vi "Main.vi"() -> ()   [LabVIEW 2019]
uses:
  <vilib>/addons/Biomedical/Controls/Biosignal/Biosignal Spectrum/Biosignal Spectrum.xctl
  <vilib>/addons/Biomedical/Biosignal Measurements/EEG/subVIs/bmt_EEG Frequency-domain Measures.ctl
  <vilib>/Simulation/Scripting/Companion Diagram/SimConfigNode/SimParams.ctl
  <vilib>/Simulation/Scripting/Companion Diagram/SimConfigNode/_simSolvers.ctl
  <vilib>/Simulation/Implementation/Shared/SIMSCR Execution Mode.ctl
  <vilib>/Simulation/Param Hierarchy/Typedefs/SIMPH Param Control Actions.ctl
  <vilib>/Simulation/Implementation/Shared/NILVSim_ParamChanged.vi
  <vilib>/Simulation/Implementation/Shared/NILVSIM_BeginStep.vi
  <vilib>/Simulation/Utility/Implementation/SIM Halt.vi
  <vilib>/Simulation/Utility/Implementation/SIM Time.vi
  <vilib>/Simulation/Implementation/Shared/SIM Is Init or Final Stage.vi
  <vilib>/Simulation/SignalDisplay/Implementation/NILVSim Time Waveform.llb/SIM Time Waveform (scalar).vi
  <vilib>/Simulation/Implementation/Shared/NILVSim_Manager.vi
  <vilib>/Utility/error.llb/Clear Errors.vi
  <vilib>/Simulation/Implementation/Shared/NILVSim_FinalizeModel.vi
  <vilib>/Simulation/Implementation/Shared/SIM Unbundle Sim Info.vi
  <vilib>/Simulation/Implementation/Shared/NILVSim_Initialize.vi
  <vilib>/Simulation/Utility/Implementation/NILVSim Get Time and IsAcceptedStep.vi
  <vilib>/Simulation/Implementation/Shared/SIMSH Read Queue.vi
  <vilib>/Simulation/Implementation/Shared/NILVSim_GetModelError.vi
  <vilib>/Simulation/Implementation/Shared/SIM Bundle Sim Info.vi
  <vilib>/Simulation/Scripting/Companion Diagram/SimConfigNode/SimDog.xnode
  <vilib>/Simulation/Implementation/XNodeFramework/SimXNode/SimX.xnode
  <vilib>/Simulation/EMI/Plugins/Multisim Design/MultisimEMICtrl.dll
  <vilib>/Simulation/Implementation/Shared/NI_SIM_Implementation.lvlib
  <vilib>/addons/Biomedical/NI_BMTK_Measurements.lvlib
panel:
  in  "Tab Control":T1(tab)
  out "Alpha Relative Power":dbl
  out "Beta Relative Power":dbl
  out "Theta Relative Power":dbl
  out "RAW EEG":dynamicdata(graph)
  in  "Halt":bool
  out "Time":dbl format="%#_3g"
  out "ACQUIRED EEG":waveform(dbl)(graph)
  in  "Tab Control 2":enum32{"Channel 1 ", "Channel 2"}(tab)
  out "Right Beta Relative Power":dbl
  out "Right Theta Relative Power":dbl
  out "Right Alpha Relative Power":dbl
  out "Right Lobe EEG":dynamicdata(graph)
  out "Right Alpha Band":waveform(dbl)[](graph)
  out "Right Beta Band":waveform(dbl)[](graph)
  out "Right Theta Band":waveform(dbl)[](graph)
  out "Left Beta Relative Power":dbl
  out "Left Alpha Relative Power":dbl
  out "Left Theta Relative Power":dbl
  out "Left Lobe EEG":dynamicdata(graph)
  out "Left Alpha Band":waveform(dbl)[](graph)
  out "Left Beta Band":waveform(dbl)[](graph)
  out "Left Theta Band":waveform(dbl)[](graph)
  in  "Tab Control 3":enum32{"Channel 1", "Channel 2"}(tab)
  out "Right Theta PSD":cluster{"f0":dbl, "df":dbl, "magnitude":dbl[]}[](graph)
  out "Right Beta PSD":cluster{"f0":dbl, "df":dbl, "magnitude":dbl[]}[](graph)
  out "Right Alpha PSD":cluster{"f0":dbl, "df":dbl, "magnitude":dbl[]}[](graph)
  out "Right Lobe EEG PSD":cluster{"f0":dbl, "df":dbl, "S(f)":dbl[]}(xcontrol)
  out "Left Theta PSD":cluster{"f0":dbl, "df":dbl, "magnitude":dbl[]}[](graph)
  out "Left Beta PSD":cluster{"f0":dbl, "df":dbl, "magnitude":dbl[]}[](graph)
  out "Left Alpha PSD":cluster{"f0":dbl, "df":dbl, "magnitude":dbl[]}[](graph)
  out "Left Lobe EEG PSD":cluster{"f0":dbl, "df":dbl, "S(f)":dbl[]}(xcontrol)
  out "?":string="Right Lobe Maximum Band"
  out "Right Beta":bool
  out "Right Alpha":bool
  out "Right Theta":bool
  out "?":string="Left Lobe Maximum Band"
  out "Left Beta":bool
  out "Left Alpha":bool
  out "Left Theta":bool
  out "Left Theta Mean (uV)":dbl format="%0.2f"
  out "Left Alpha Mean (uV)":dbl format="%0.2f"
  out "Left Beta Mean (uV)":dbl format="%0.2f"
  out "Right Theta Mean (uV)":dbl format="%0.2f"
  out "Right Alpha Mean (uV)":dbl format="%0.2f"
  out "Right Beta Mean (uV)":dbl format="%0.2f"
  out "Left Lobe  (uV^2)":T2 {"beta [%]" format="%_3g"; "alpha [%]" format="%_3g"; "theta [%]" format="%_3g"; "delta [%]" format="%_3g"; "beta power" format="%_3g"; "alpha power" format="%_3g"; "theta power" format="%_3g"; "delta power" format="%_3g"}
  out "Right Lobe  (uV^2)":T2 {"beta [%]" format="%_3g"; "alpha [%]" format="%_3g"; "theta [%]" format="%_3g"; "delta [%]" format="%_3g"; "beta power" format="%_3g"; "alpha power" format="%_3g"; "theta power" format="%_3g"; "delta power" format="%_3g"}
  out "?":string
  out "Left Frontal Lobe":bool
  out "Right Frontal Lobe":bool
  out "Veredict":string
  # "EEG in a perspective of hemispherical frontal asymmetry: Mean value of alpha wave from the left frontal lobe is compared with that of the right frontal lobe.\nIf the signal from the left is stronger, there is an indication that the participant is especially interested and motivated at a precise moment of decision making during the completion of a task."
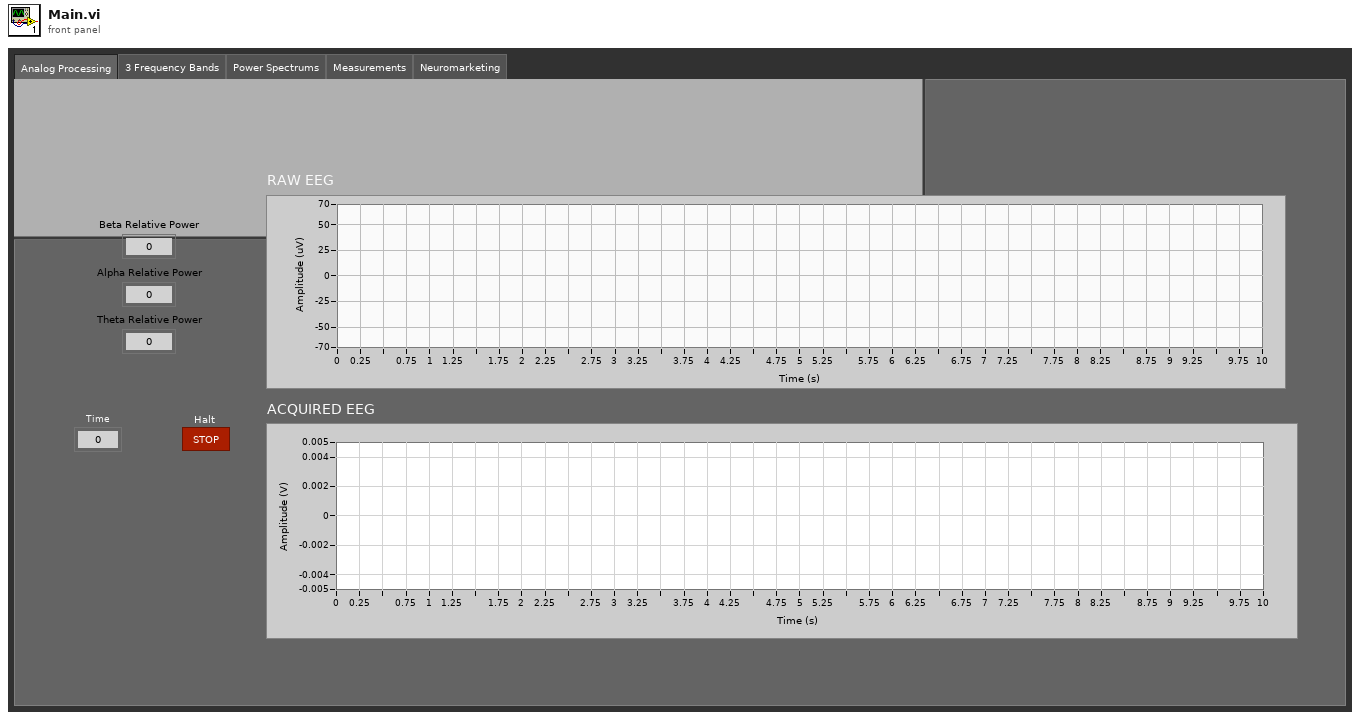
[diagram p1: front panel]
types:
  T1 = enum32{"Analog Processing", "3 Frequency Bands", "Power Spectrums", "Measurements", "Neuromarketing"}
  T2 = typedef "NI_BMTK_Measurements.lvlib/bmt_EEG Frequency-domain Measures.ctl" = cluster{"delta power":dbl, "theta power":dbl, "alpha power":dbl, "beta power":dbl, "delta [%]":dbl, "theta [%]":dbl, "alpha [%]":dbl, "beta [%]":dbl}
  T3 = typedef "SIMSCR Execution Mode.ctl" = enum16{"Simulate to Completion", "Single Time-Step Simulation (Fixed Step Only)"}
  T4 = typedef "SIMPH Param Control Actions.ctl" = enum16{"get params", "set params"}
  T5 = typedef "SimParams.ctl" = cluster{"Initial Time (s)":dbl, "Final Time (s)":dbl, "Step Size (s)":dbl, "ODE Solver":T6, "Minimum Step Size (s)":dbl, "Maximum Step Size (s)":dbl, "Relative Tolerance":dbl, "Absolute Tolerance":dbl, "Software Timing":bool, "Initial Step Size (s)":dbl, "Automatic Fixed Step Size?":bool, "Automatic Discrete Step Size?":bool, "Discrete Step Size (s)":dbl, "Calculate using Time Step":bool, "Solver Wired?":bool, "Prev.Frm.Expected End":u64, "Prev.Frm.Actual End":u64, "Prev.Frm.Finished Late?":bool, "Prev.Iter.Expected End":u64, "Prev.Iter.Actual End":u64, "Prev.Iter.Finished Late?":bool, "Expected Iteration Start":u64, "Actual Iteration Start":u64, "Expected Frame Start":u64, "Actual Frame Start":u64, "Source Name":string, "Name":string, "Period":i64, "Deadline":i64, "Offset":i64, "Start":i64, "Priority":i32, "Timeout":i32, "Processor":i32, "Mode":enum32{"No Change", "Process missed periods, maintain original phase", "Discard missed periods, maintain original phase", "Process missed periods, ignore original phase", "Discard missed periods, ignore original phase"}, "Wakeup reason":enum32{"Normal", "Aborted", "Asynchronous wakeup", "Timing source error", "Timed loop error", "Timeout"}, "Error":errorcluster, "Source Type":string, "Secondary Source Type":string, "Global End Time":u64, "Global Start Time":u64, "Full Solver Reset":bool, "Execution Mode":T3, "Nan/Inf Check":bool, "Custom Solver Library":string, "Solver Is Variable":bool, "custom solver name":string, "Signal Collection Decimation":u32}
  T6 = typedef "_simSolvers.ctl" = enum16{"Runge-Kutta 1 (Euler)", "Runge-Kutta 2", "Runge-Kutta 3", "Runge-Kutta 4", "Runge-Kutta 23 (variable)", "Runge-Kutta 45 (variable)", "BDF (variable)", "Adams-Moulton (variable)", "Rosenbrock (variable)", "Discrete States Only", "SDIRK 4 (variable)", "Radau 5 (variable)", "Radau 9 (variable)", "Radau 13 (variable)", "Radau [Variable Order] (variable)", "Gear's Method (variable)", "Linearizer", "State Query", "Trim Eval", "Custom Solver"}
  T7 = cluster{"Topology":enum16{"Off", "Butterworth", "Chebyshev", "Inverse Chebyshev", "Elliptic", "Bessel"}, "Type":enum16{"Lowpass", "Highpass", "Bandpass", "Bandstop"}, "Order":i32, "Lower Fc":dbl, "Upper Fc":dbl, "PB Ripple":dbl, "SB Attenuation":dbl}
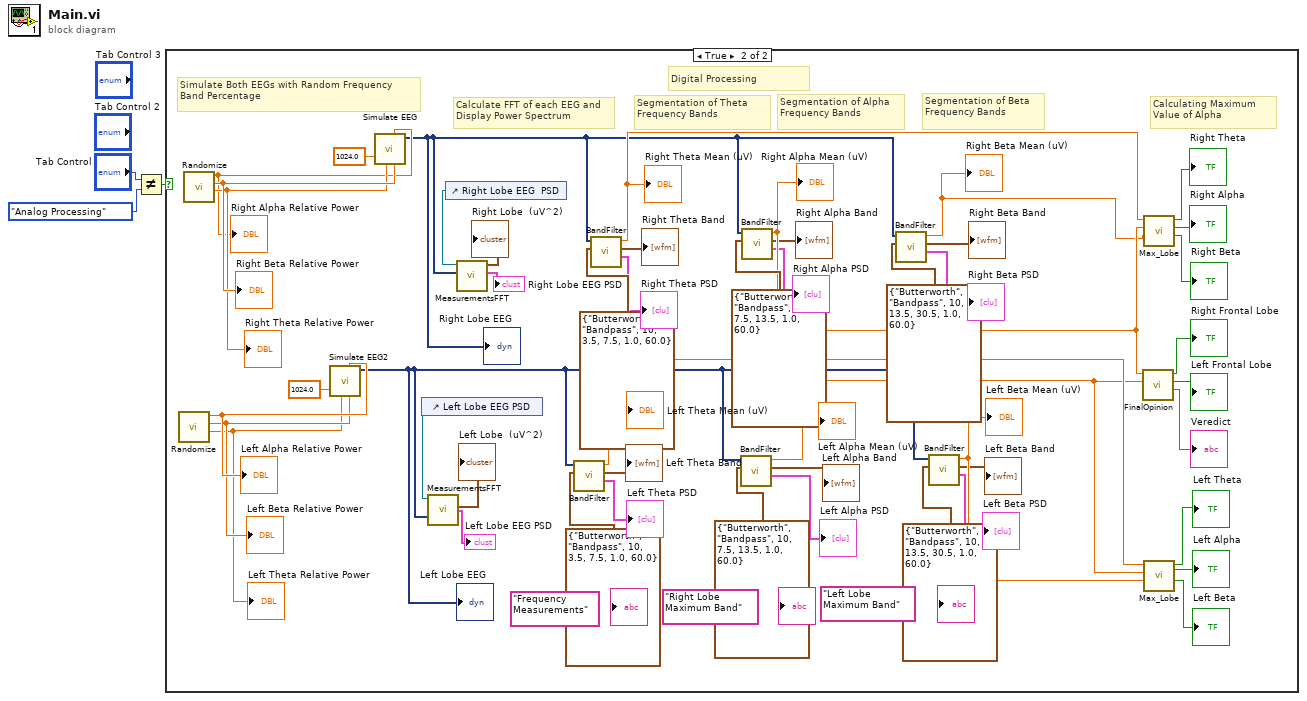
[diagram p0: block diagram]
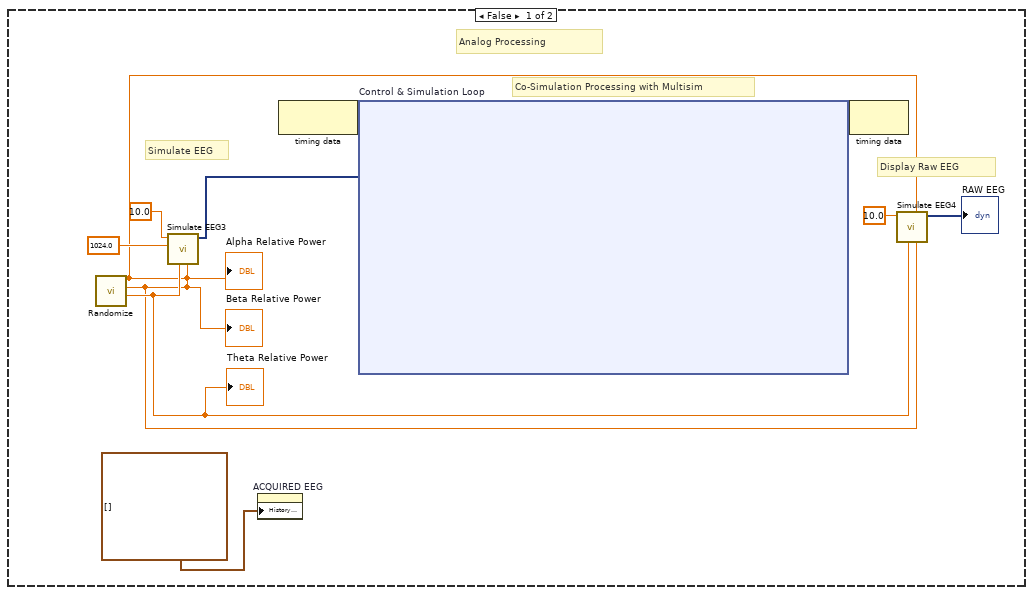
[diagram p2: hidden frame]
diagram:
  n1 = Not Equal?(x="Tab Control", y=T1."Analog Processing") -> (x != y?=w1:bool)
  n2 = case shown="True" w1 {
    frame False {
      # "Display Raw EEG"
      # "Co-Simulation Processing with Multisim"
      # "Simulate EEG"
      # "Analog Processing"
      n3 = call "Randomize.vi"() -> ("Theta"=w6:dbl, "Beta"=w5:dbl, "Alpha"=w4:dbl)  [unwired: 9 in]
      "Alpha Relative Power" <- w4
      "Beta Relative Power" <- w5
      "Theta Relative Power" <- w6
      n4 = call "Simulate EEG3"("power_beta"=w5, "power_alpha"=w4, "power_theta"=w6, "sampling rate"=1024.0, "block size"=10.0) -> ("EEG"=w9:dynamicdata)  [unwired: 5 in, 1 out]
      n5 = property on="ACQUIRED EEG" class="WFChart (strict)"("History Data"=waveform(dbl)[] []) -> ()  [unwired: 2 in, 2 out]
      n6 = node-c288() -> (w14:variant)  [unwired: 1 in]
      n7 = node-c254 "Control & Simulation Loop"(w14, w9) -> (w13:variant)
      n8 = node-c288(w13) -> ()  [unwired: 1 out]
      n9 = call "Simulate EEG4"("power_beta"=w5, "power_alpha"=w4, "power_theta"=w6, "block size"=10.0) -> ("EEG"=→"RAW EEG":dynamicdata)  [unwired: 6 in, 1 out]
    }
    frame True {
      # "Calculating Maximum Value of Alpha"
      # "Calculate FFT of each EEG and Display Power Spectrum"
      # "Segmentation of Beta Frequency Bands"
      # "Segmentation of Alpha Frequency Bands"
      # "Segmentation of Theta Frequency Bands"
      # "Simulate Both EEGs with Random Frequency Band Percentage"
      # "Digital Processing"
      n10 = call "Randomize.vi"() -> ("Theta"=w344:dbl, "Beta"=w345:dbl, "Alpha"=w346:dbl)  [unwired: 9 in]
      "Left Alpha Relative Power" <- w346
      "Left Beta Relative Power" <- w345
      "Left Theta Relative Power" <- w344
      n11 = call "Randomize.vi"() -> ("Theta"=w347:dbl, "Beta"=w348:dbl, "Alpha"=w318:dbl)  [unwired: 9 in]
      "Right Alpha Relative Power" <- w318
      "Right Beta Relative Power" <- w348
      "Right Theta Relative Power" <- w347
      n12 = call "Simulate EEG2"("power_beta"=w345, "power_alpha"=w346, "power_theta"=w344, "sampling rate"=1024.0) -> ("EEG"=w322:dynamicdata)  [unwired: 6 in, 1 out]
      "Left Lobe EEG" <- w322
      n13 = call "Simulate EEG"("power_beta"=w348, "power_alpha"=w318, "power_theta"=w347, "sampling rate"=1024.0) -> ("EEG"=w317:dynamicdata)  [unwired: 6 in, 1 out]
      "Right Lobe EEG" <- w317
      n14 = control-ref of="Left Lobe EEG PSD"() -> (w357:refnum<vi>)
      n15 = call "MeasurementsFFT.vi"("Left Lobe EEG"=w322, "Control in"=w357) -> ("Spectrum Out"=→"Left Lobe EEG PSD":cluster{"f0":dbl, "df":dbl, "S(f)":dbl[]}, "Frequency Measurements"=→"Left Lobe  (uV^2)":T2)  [unwired: 8 in]
      n16 = control-ref of="Right Lobe EEG  PSD"() -> (w354:refnum<vi>)
      n17 = call "MeasurementsFFT.vi"("Left Lobe EEG"=w317, "Control in"=w354) -> ("Spectrum Out"=→"Right Lobe EEG PSD":cluster{"f0":dbl, "df":dbl, "S(f)":dbl[]}, "Frequency Measurements"=→"Right Lobe  (uV^2)":T2)  [unwired: 8 in]
      n18 = call "BandFilter.vi"("IIR filter specifications"=T7 {"Topology"=enum."Butterworth", "Type"=enum."Bandpass", "Order"=10, "Lower Fc"=3.5, "Upper Fc"=7.5, "PB Ripple"=1.0, "SB Attenuation"=60.0}, "Right Lobe EEG"=w322) -> ("PSD"=→"Left Theta PSD":cluster{"f0":dbl, "df":dbl, "magnitude":dbl[]}[], "signal(s) out"=→"Left Theta Band":waveform(dbl)[], "mean"=w330:dbl)  [unwired: 7 in]
      "Left Theta Mean (uV)" <- w330
      n19 = call "BandFilter.vi"("IIR filter specifications"=T7 {"Topology"=enum."Butterworth", "Type"=enum."Bandpass", "Order"=10, "Lower Fc"=3.5, "Upper Fc"=7.5, "PB Ripple"=1.0, "SB Attenuation"=60.0}, "Right Lobe EEG"=w317) -> ("PSD"=→"Right Theta PSD":cluster{"f0":dbl, "df":dbl, "magnitude":dbl[]}[], "signal(s) out"=→"Right Theta Band":waveform(dbl)[], "mean"=w342:dbl)  [unwired: 7 in]
      "Right Theta Mean (uV)" <- w342
      n20 = call "BandFilter.vi"("IIR filter specifications"=T7 {"Topology"=enum."Butterworth", "Type"=enum."Bandpass", "Order"=10, "Lower Fc"=7.5, "Upper Fc"=13.5, "PB Ripple"=1.0, "SB Attenuation"=60.0}, "Right Lobe EEG"=w322) -> ("PSD"=→"Left Alpha PSD":cluster{"f0":dbl, "df":dbl, "magnitude":dbl[]}[], "signal(s) out"=→"Left Alpha Band":waveform(dbl)[], "mean"=w326:dbl)  [unwired: 7 in]
      "Left Alpha Mean (uV)" <- w326
      n21 = call "BandFilter.vi"("IIR filter specifications"=T7 {"Topology"=enum."Butterworth", "Type"=enum."Bandpass", "Order"=10, "Lower Fc"=7.5, "Upper Fc"=13.5, "PB Ripple"=1.0, "SB Attenuation"=60.0}, "Right Lobe EEG"=w317) -> ("PSD"=→"Right Alpha PSD":cluster{"f0":dbl, "df":dbl, "magnitude":dbl[]}[], "signal(s) out"=→"Right Alpha Band":waveform(dbl)[], "mean"=w338:dbl)  [unwired: 7 in]
      "Right Alpha Mean (uV)" <- w338
      n22 = call "BandFilter.vi"("IIR filter specifications"=T7 {"Topology"=enum."Butterworth", "Type"=enum."Bandpass", "Order"=10, "Lower Fc"=13.5, "Upper Fc"=30.5, "PB Ripple"=1.0, "SB Attenuation"=60.0}, "Right Lobe EEG"=w317) -> ("PSD"=→"Right Beta PSD":cluster{"f0":dbl, "df":dbl, "magnitude":dbl[]}[], "signal(s) out"=→"Right Beta Band":waveform(dbl)[], "mean"=w334:dbl)  [unwired: 7 in]
      "Right Beta Mean (uV)" <- w334
      n23 = call "BandFilter.vi"("IIR filter specifications"=T7 {"Topology"=enum."Butterworth", "Type"=enum."Bandpass", "Order"=10, "Lower Fc"=13.5, "Upper Fc"=30.5, "PB Ripple"=1.0, "SB Attenuation"=60.0}, "Right Lobe EEG"=w322) -> ("PSD"=→"Left Beta PSD":cluster{"f0":dbl, "df":dbl, "magnitude":dbl[]}[], "signal(s) out"=→"Left Beta Band":waveform(dbl)[], "mean"=w321:dbl)  [unwired: 7 in]
      "Left Beta Mean (uV)" <- w321
      n24 = call "FinalOpinion.vi"("Left Alpha Mean"=w326, "Right Alpha Mean"=w338) -> ("Decision"=→"Veredict":string, "Left Higher"=→"Left Frontal Lobe":bool, "Right Higher"=→"Right Frontal Lobe":bool)  [unwired: 7 in]
      n25 = call "Max_Lobe.vi"("Beta Mean"=w334, "Alpha Mean"=w338, "Theta Mean"=w342) -> ("Beta"=→"Right Beta":bool, "Alpha"=→"Right Alpha":bool, "Theta"=→"Right Theta":bool)  [unwired: 6 in]
      n26 = call "Max_Lobe.vi"("Beta Mean"=w321, "Alpha Mean"=w326, "Theta Mean"=w330) -> ("Beta"=→"Left Beta":bool, "Alpha"=→"Left Alpha":bool, "Theta"=→"Left Theta":bool)  [unwired: 6 in]
      "?" <- "Frequency Measurements"
      "?" <- "Left Lobe Maximum Band"
      "?" <- "Right Lobe Maximum Band"
    }
  }
